vi "Speed Sensitivity.vi"(8 "Tuning":T1={"Max Speed"=1.0, "Min Speed"=0.35, "Deadzone"=0.1} {"Deadzone" min=0.0 max=1.0; "Min Speed" min=0.0 max=1.0; "Max Speed" min=0.0 max=1.0}, 11 "Input":dbl) -> (3 "Output":dbl)   [LabVIEW 2017]
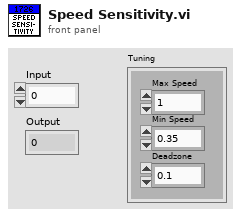
[diagram p1: front panel]
types:
  T1 = cluster{"Max Speed":dbl, "Min Speed":dbl, "Deadzone":dbl}
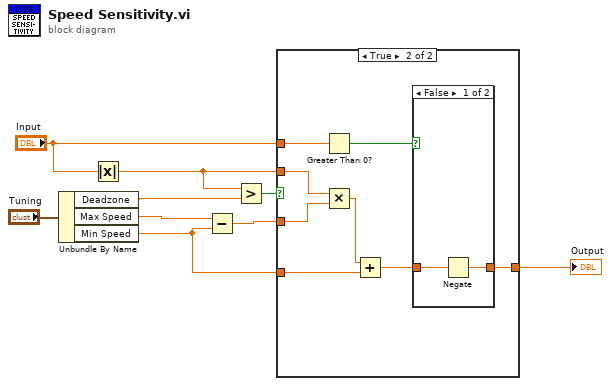
[diagram p0: block diagram]
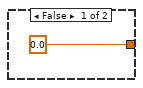
[diagram p2: hidden frame]
diagram:
  n1 = Unbundle By Name("Tuning") -> ("Deadzone"=w1:dbl, "Max Speed"=w3:dbl, "Min Speed"=w2:dbl)
  n2 = Absolute Value(x="Input") -> (abs(x)=w7:dbl)
  n3 = Subtract(x=w3, y=w2) -> (x-y=w5:dbl)
  n4 = Greater?(x=w7, y=w1) -> (0:w9:bool)
  n5 = case shown="True" w9 {
    tunnel: [0.0 w15] -> w8
    tunnel: w7 -> [_ w18]
    tunnel: "Input" -> [_ w13]
    tunnel: w5 -> [_ w12]
    tunnel: w2 -> [_ w11]
    frame False {
    }
    frame True {
      n6 = Greater Than 0?(x=w13) -> (x > 0?=w14:bool)
      n7 = Multiply(x=w18, y=w12) -> (x*y=w17:dbl)
      n8 = Add(x=w17, y=w11) -> (x+y=w16:dbl)
      n9 = case shown="False" w14 {
        tunnel: w16 -> [w20 w21]
        tunnel: [w19 w21] -> w15
        frame False {
          n10 = Negate(x=w20) -> (-x=w19:dbl)
        }
        frame True {
        }
      }
    }
  }
  "Output" <- w8
